vi "Uframe-Motor_Cal.vi"() -> ()   [LabVIEW 2010]
uses:
  <vilib>/Platform/TimedLoop/XDataNode/XDataNode.xnode
  <vilib>/Platform/TimedLoop/XDataNode/timing_clust.ctl
  <vilib>/Platform/TimedLoop/XDataNode/nitl_modes.ctl
  <vilib>/Platform/TimedLoop/XDataNode/wakeup.ctl
  <vilib>/Platform/TimedLoop/XDataNode/XDNodeRunTimeDep.lvlib
panel:
  in  "Duty Cycle":dbl min=0.0 max=100.0 step=5.0
  out "Numeric":i32
  in  "Invert Disp":bool
  in  "Zero Displacement":bool
  in  "Begin":bool
  in  "Stop":bool
  out "Disp Vs Time":cluster{dbl[], dbl[]}(graph)={[-724.1250113144533, -724.195323815552, -724.2656363166506, -724.3359488177492, -724.4062613188479, -724.4765738199465, -724.5468863210451, -724.6171988221438, -724.7461050741579, -724.9218863269045, -725.0976675796511, -725.2851675825808, -725.4492300851442], [-11.89350874713131, -11.896152101474941, -11.894229661847117, -11.89350874707076, -11.890865392620372, -11.895671491596438, -11.895911796524977, -11.899756675680168, -11.899035760801853, -11.90552399441818, -11.907927043887174, -11.905283689458143, -11.914655582386047]}
  in  "File Name":string="Test"
  in  "File Path":path=path "C:/cygwin/home/Smarter Materials/Users 2015/Michael Rossol"
  in  "Sample Notes":string
  in  "Data Acquisition Interval (s)":dbl min=0.01 max=60.0 step=0.01
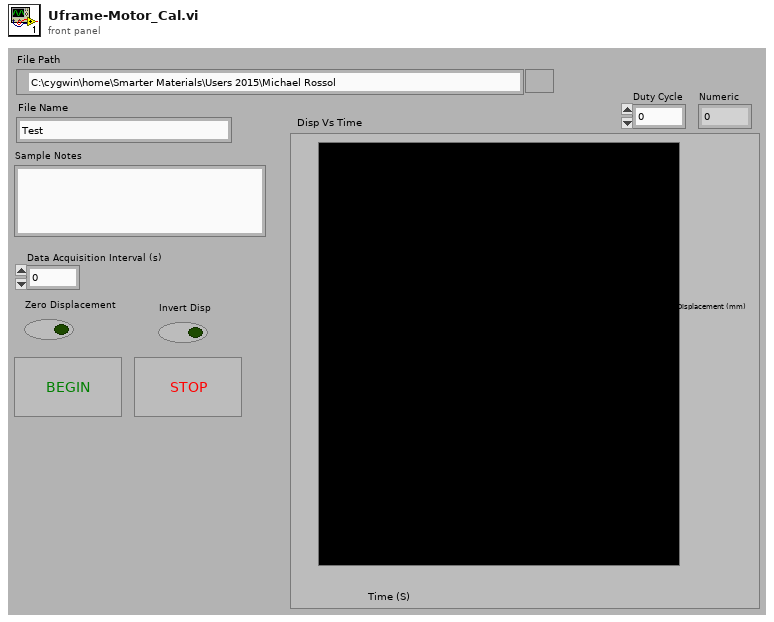
[diagram p1: front panel]
types:
  T1 = typedef "XDNodeRunTimeDep.lvlib/timing_clust.ctl" = cluster{"Expected End [f-1]":u64, "Actual End [f-1]":u64, "Finished Late? [f-1]":bool, "Expected End [i-1]":u64, "Actual End [i-1]":u64, "Finished Late? [i-1]":bool, "Expected Start [i]":u64, "Actual Start [i]":u64, "Expected Start [f]":u64, "Actual Start [f]":u64, "Source Name":string, "Structure Name":string, "Period":i64, "Deadline":i64, "Offset":i64, "Start":i64, "Priority":i32, "Timeout":i32, "Mode":T2, "Wakeup Reason":T3, "Error":errorcluster, "Source Type":string, "Secondary Source Type":string, "Global End Time":u64, "Global Start Time":u64, "Frame Duration":u64, "Iteration Duration":u64, "Assigned CPU":i32, "I/O Scan Engine Mode":u32}
  T2 = typedef "XDNodeRunTimeDep.lvlib/nitl_modes.ctl" = enum32{"No Change", "Process missed periods, maintain original phase", "Discard missed periods, maintain original phase", "Process missed periods, ignore original phase", "Discard missed periods, ignore original phase"}
  T3 = typedef "XDNodeRunTimeDep.lvlib/wakeup.ctl" = enum32{"Normal", "Aborted", "Asynchronous wakeup", "Timing source error", "Timed loop error", "Timeout"}
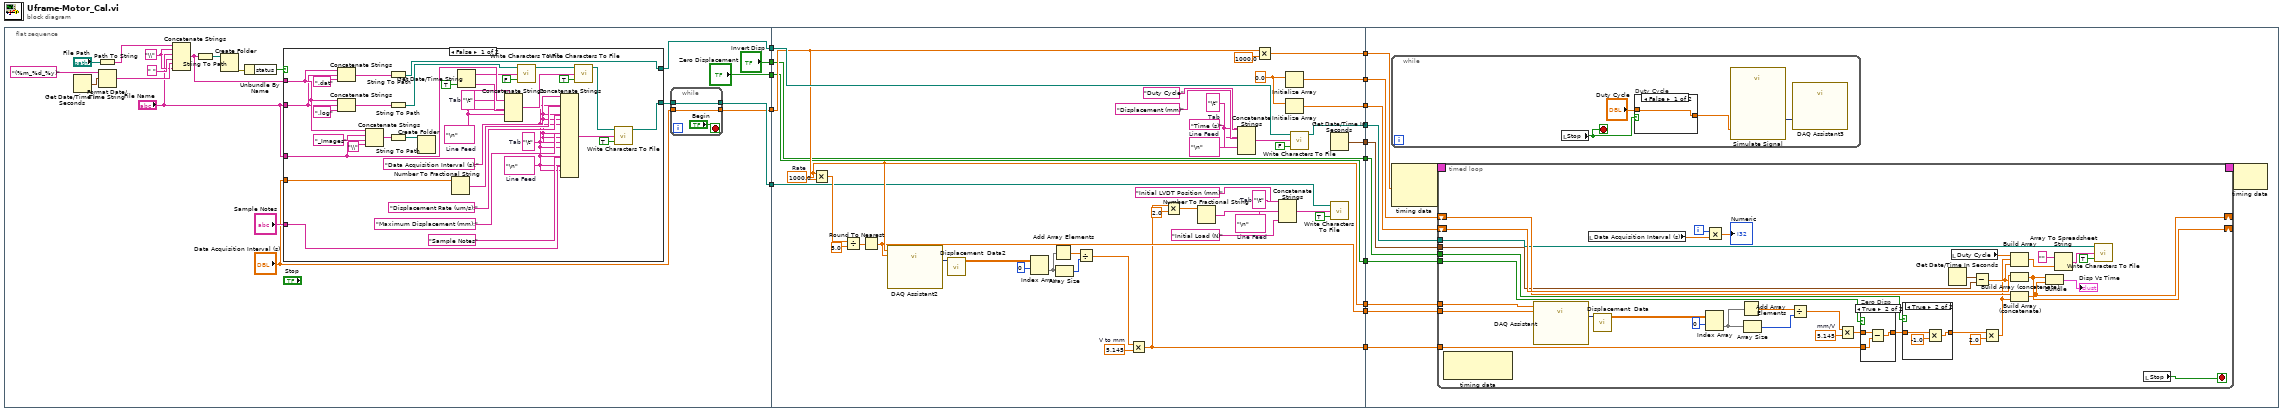
[diagram p0: block diagram]
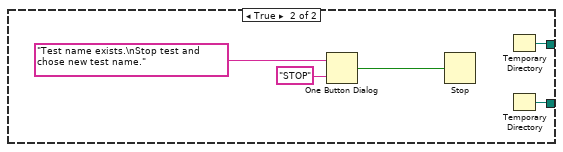
[diagram p2: hidden frame]
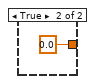
[diagram p3: hidden frame]
diagram:
  n1 = flat-sequence {
    tunnel: [w21] -> w8
    tunnel: [w20] -> w6
    tunnel: [w19] -> w5
    tunnel: ["Zero Displacement"] -> w3
    tunnel: ["Invert Disp"] -> w2
    tunnel: [w107] -> w15
    tunnel: [w106] -> w14
    tunnel: [w105] -> w13
    tunnel: [w104] -> w12
    tunnel: [w103] -> w11
    tunnel: [w80] -> w10
    tunnel: [w95] -> w9
    tunnel: w8 -> [w94]
    tunnel: [w89] -> w7
    tunnel: w6 -> [w88]
    tunnel: w5 -> [w87]
    tunnel: [w86] -> w4
    tunnel: w3 -> [w86]
    tunnel: w2 -> [w85]
    tunnel: [w85] -> w1
    tunnel: w15 -> [w130]
    tunnel: w14 -> [w129]
    tunnel: w13 -> [w128]
    tunnel: w12 -> [w127]
    tunnel: w11 -> [w126]
    tunnel: w10 -> [w125]
    tunnel: w9 -> [w124]
    tunnel: w7 -> [w123]
    tunnel: w4 -> [w122]
    tunnel: w1 -> [w121]
    frame #0 {
      w29 = "\\"
      n2 = Get Date/Time In Seconds() -> (seconds since 1Jan1904=w32:timestamp)
      n3 = Path To String(path="File Path") -> (string=w35:string)
      n4 = Format Date/Time String(time format string (%c)="(%m_%d_%y)", seconds (now)=w32) -> (date/time string=w31:string)  [unwired: 1 in]
      n5 = Concatenate Strings(w35, w29, "File Name", " ", w31, w29) -> (w24:string)
      n6 = String To Path(string=w24) -> (path=w28:path)
      n7 = Create Folder(path (use dialog)=w28) -> (error out=w34:errorcluster)  [unwired: 2 in, 2 out]
      n8 = Unbundle By Name(w34) -> ("status"=w27:bool)
      n9 = case shown="False" w27 {
        tunnel: w24 -> [w41 _]
        tunnel: "File Name" -> [w40 _]
        tunnel: [w46 w75] -> w22
        tunnel: "File Name" -> [w45 _]
        tunnel: "Data Acquisition Interval (s)" -> [w61 _]
        tunnel: "Sample Notes" -> [w48 _]
        tunnel: [w42 w74] -> w20
        frame False {
          w39 = "\t"  # Tab
          w47 = "\n"  # Line Feed
          w64 = "\t"  # Tab
          w58 = "\n"  # Line Feed
          n10 = Concatenate Strings(w41, w40, ".dat") -> (w43:string)
          n11 = Concatenate Strings(w41, w40, ".log") -> (w66:string)
          n12 = Concatenate Strings(w41, w45, "_Images", "\\") -> (w54:string)
          n13 = String To Path(string=w43) -> (path=w42:path)
          n14 = String To Path(string=w66) -> (path=w71:path)
          n15 = String To Path(string=w54) -> (path=w53:path)
          n16 = Create Folder(path (use dialog)=w53) -> ()  [unwired: 2 in, 3 out]
          n17 = Number To Fractional String(number=w61) -> (F-format string=w52:string)  [unwired: 3 in]
          n18 = Get Date/Time String(want seconds? (F)=TRUE) -> (date string=w69:string, time string=w68:string)  [unwired: 2 in]
          n19 = Concatenate Strings(w58, w69, w64, w68, w58, w58) -> (w70:string)
          n20 = call <vilib>:"Write Characters To File.vi"("append to file? (new file:F)"=FALSE, "character string"=w45, "file path (dialog if empty)"=w71) -> ("new file path (Not A Path if cancelled)"=w67:path)  [unwired: 2 in]
          n21 = Concatenate Strings("Data Acquisition Interval (s):", w39, w52, w47, "Displacement Rate (um/s):", w39, w39, w47, "Maximum Displacement (mm):", w39, w39, w47, w47, "Sample Notes", w47, w48, w47, w47) -> (w59:string)
          n22 = call <vilib>:"Write Characters To File.vi"("append to file? (new file:F)"=TRUE, "character string"=w70, "file path (dialog if empty)"=w67) -> ("new file path (Not A Path if cancelled)"=w62:path)  [unwired: 2 in]
          n23 = call <vilib>:"Write Characters To File.vi"("append to file? (new file:F)"=TRUE, "character string"=w59, "file path (dialog if empty)"=w62) -> ("new file path (Not A Path if cancelled)"=w46:path)  [unwired: 2 in]
        }
        frame True {
          n24 = One Button Dialog(message="Test name exists.\nStop test and chose new test name.", button name ("OK")="STOP") -> (true=w76:bool)
          n25 = Stop(stop? (T)=w76) -> ()
          n26 = Temporary Directory() -> (w74:path)
          n27 = Temporary Directory() -> (w75:path)
        }
      }
      n28 = while {
        tunnel: [w38] -> w21
        tunnel: w22 -> [w38]
        tunnel: [w36] -> w19
        tunnel: "Data Acquisition Interval (s)" -> [w36]
        stop <- "Begin" stop-if-true
      }
    }
    frame #1 {
      w82 = "\n"  # Line Feed
      w83 = "\t"  # Tab
      w99 = "\n"  # Line Feed
      w97 = "\t"  # Tab
      w115 = 5.145  # V to mm
      w104 = 1000.0  # Rate
      w119 = 0.0
      n29 = Multiply(x=w104, y=w87) -> (x*y=w118:dbl)
      n30 = Divide(x=w118, y=5.0) -> (x/y=w116:dbl)
      n31 = Round To Nearest(number=w116) -> (nearest integer value=w103:dbl)
      n32 = call "DAQ Assistant2"("rate"=w104, "number of samples"=w103) -> ("data"=w108:dynamicdata)  [unwired: 15 in, 2 out]
      n33 = call "Displacement  Data2"("Dynamic Data Type"=w108) -> ("Array"=w110:dbl[][])  [unwired: 3 in]
      n34 = Index Array(array=w110, index (row)=0) -> (element=w111:dbl[])  [unwired: 1 in]
      n35 = Add Array Elements(numeric array=w111) -> (sum=w112:dbl)
      n36 = Array Size(array=w111) -> (size(s)=w113:i32)
      n37 = Divide(x=w112, y=w113) -> (x/y=w114:dbl)
      n38 = Multiply(x=w114, y=w115) -> (x*y=w80:dbl)
      n39 = Multiply(x=w80, y=2.0) -> (x*y=w81:dbl)
      n40 = Number To Fractional String(number=w81) -> (F-format string=w98:string)  [unwired: 3 in]
      n41 = Concatenate Strings("Duty Cycle", w83, "Displacement (mm)" ("Substring"), w83, "Time (s)" ("string"), w82) -> (w92:string)
      n42 = Multiply(x=w87, y=1000.0) -> (x*y=w107:dbl)
      n43 = Concatenate Strings("Initial LVDT Position (mm)", w97, w98, w99, "Initial Load (N)") -> (w101:string)
      n44 = Initialize Array(w119) -> (w106:dbl[])  [unwired: 1 in]
      n45 = Initialize Array(w119) -> (w105:dbl[])  [unwired: 1 in]
      n46 = call <vilib>:"Write Characters To File.vi"("append to file? (new file:F)"=FALSE, "character string"=w92, "file path (dialog if empty)"=w88) -> ("new file path (Not A Path if cancelled)"=w89:path)  [unwired: 2 in]
      n47 = Get Date/Time In Seconds() -> (seconds since 1Jan1904=w95:timestamp)
      n48 = call <vilib>:"Write Characters To File.vi"("append to file? (new file:F)"=TRUE, "character string"=w101, "file path (dialog if empty)"=w94) -> ()  [unwired: 2 in, 1 out]
    }
    frame #2 {
      n49 = while {
        stop <- w135 stop-if-true
        n50 = local read "Stop"() -> (w135:bool)
        n51 = case "Duty Cycle" shown="False" w135 {
          tunnel: [w137 0.0 ("Duty Cycle (%)")] -> w134
          tunnel: "Duty Cycle" -> [w137 _]
          frame False {
          }
          frame True {
          }
        }
        n52 = call "Simulate Signal"("Duty Cycle (%)"=w134) -> ("Square"=w136:dynamicdata)  [unwired: 13 in, 1 out]
        n53 = call "DAQ Assistant3"("data"=w136) -> ()  [unwired: 16 in, 3 out]
      }
      n54 = node-c288 ("Input Node")(w130) -> (w132:T1)  [unwired: 2 in]
      n55 = timed-loop {
        shift-left: w129 -> [w157]
        shift-right: [w148] -> _
        shift-left: w128 -> [w158]
        shift-right: [w149] -> _
        timing-out: [_] -> w131
        timing: w132 -> [_]
        tunnel: w126 -> [w163]
        tunnel: w127 -> [w162]
        tunnel: w125 -> [w154]
        tunnel: w124 -> [w156]
        tunnel: w123 -> [w155]
        tunnel: w122 -> [w152]
        tunnel: w121 -> [w150]
        i -> [w143]
        stop <- w145 stop-if-true
        w161 = 5.145  # mm/V
        n56 = node-c288() -> ()  [unwired: 1 in, 2 out]
        n57 = call "DAQ Assistant"("rate"=w162, "number of samples"=w163) -> ("data"=w160:dynamicdata)  [unwired: 15 in, 2 out]
        n58 = local read "Data Acquisition Interval (s)"() -> (w144:dbl)
        n59 = call "Displacement  Data"("Dynamic Data Type"=w160) -> ("Array"=w169:dbl[][])  [unwired: 3 in]
        n60 = Index Array(array=w169, index (row)=0) -> (element=w167:dbl[])  [unwired: 1 in]
        n61 = Multiply(x=w143, y=w144) -> (x*y=→"Numeric":dbl)
        n62 = Add Array Elements(numeric array=w167) -> (sum=w166:dbl)
        n63 = Array Size(array=w167) -> (size(s)=w165:i32)
        n64 = Divide(x=w166, y=w165) -> (x/y=w164:dbl)
        n65 = Multiply(x=w164, y=w161) -> (x*y=w153:dbl)
        n66 = case "Zero Disp" shown="True" w152 {
          tunnel: w154 -> [_ w182]
          tunnel: w153 -> [w179 w181]
          tunnel: [w179 w180] -> w151
          frame False {
          }
          frame True {
            n67 = Subtract(x=w181, y=w182) -> (x-y=w180:dbl)
          }
        }
        n68 = case shown="True" w150 {
          tunnel: w151 -> [w175 w178]
          tunnel: [w175 w177] -> w140
          frame False {
          }
          frame True {
            n69 = Multiply(x=w178, y=-1.0) -> (x*y=w177:dbl)
          }
        }
        n70 = Get Date/Time In Seconds() -> (seconds since 1Jan1904=w168:timestamp)
        n71 = local read "Duty Cycle"() -> (w146:dbl)
        n72 = Subtract(x=w168, y=w156) -> (x-y=w147:dbl)
        n73 = Multiply(x=w140, y=2.0) -> (x*y=w141:dbl)
        n74 = Build Array(w146, w141, w147) -> (w171:dbl[])
        n75 = Build Array (concatenate)(w158, w147) -> (w149:dbl[])
        n76 = Build Array (concatenate)(w157, w141) -> (w148:dbl[])
        n77 = Bundle(w149, w148) -> (→"Disp Vs Time":cluster{dbl[], dbl[]})  [unwired: 1 in]
        n78 = Array To Spreadsheet String(array=w171, 3:"" ("format string")) -> (spreadsheet string=w173:string)  [unwired: 1 in]
        n79 = call <vilib>:"Write Characters To File.vi"("append to file? (new file:F)"=TRUE, "character string"=w173, "file path (dialog if empty)"=w155) -> ()  [unwired: 2 in, 1 out]
        n80 = local read "Stop"() -> (w145:bool)
      }
      n81 = node-c288(w131) -> ()  [unwired: 1 out]
    }
  }
